vi "FreqMM.vi"(0 "measurement method":i32) -> (1 "meastime vis":bool, 2 "divisor vis":bool)   [LabVIEW 2010]
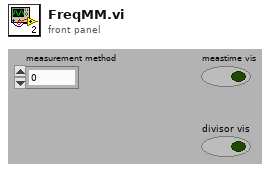
[diagram p1: front panel]
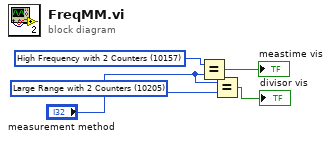
[diagram p0: block diagram]
diagram:
  w4 = 10205 items=["Low Frequency with 1 Counter"=10105, "High Frequency with 2 Counters"=10157, "Large Range with 2 Counters"=10205] ("measurement method")
  w1 = 10157 items=["Low Frequency with 1 Counter"=10105, "High Frequency with 2 Counters"=10157, "Large Range with 2 Counters"=10205] ("measurement method")
  n1 = Equal?(x=w1, y="measurement method") -> (x = y?=→"meastime vis":bool)
  n2 = Equal?(x="measurement method", y=w4) -> (x = y?=→"divisor vis":bool)
